vi "Insight_Upgrade.vi"(8 "error in (no error)":errorcluster, 9 "filename":string="?", 10 "Mode (Read / Write)":enum8{"Write", "Read"}(ring), 11 "telnet connection":T1) -> (0 "error out":errorcluster, 1 "upgrade files":string[](array[string]), 2 "response data":string, 3 "telnet  connection out":T1)   [LabVIEW 2015]
uses:
  Telnet Session.ctl
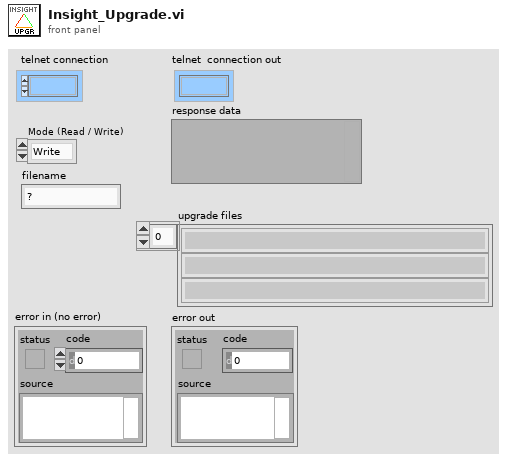
[diagram p1: front panel]
types:
  T1 = typedef "Telnet Session.ctl" = refnum<k1>
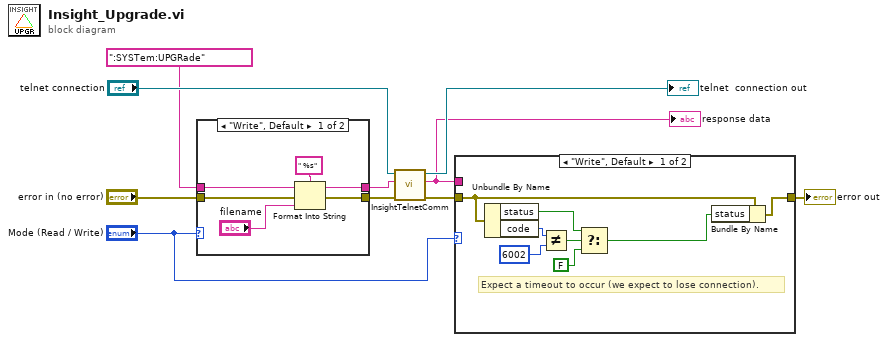
[diagram p0: block diagram]
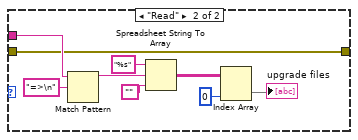
[diagram p2: hidden frame]
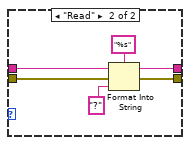
[diagram p3: hidden frame]
diagram:
  n1 = case shown="\"Write\", Default" "Mode (Read / Write)" {
    tunnel: [w12 w18] -> w6
    tunnel: "error in (no error)" -> [w13 w17]
    tunnel: ":SYSTem:UPGRade" ("String") -> [w15 w20]
    tunnel: [w14 w19] -> w5
    frame "Write", Default {
      n2 = Format Into String(format string=" %s", initial string=w15, error in=w13, "filename") -> (resulting string=w14:string, error out=w12:errorcluster)
    }
    frame "Read" {
      n3 = Format Into String(format string="%s", initial string=w20, error in=w17, "?" ("input 1")) -> (resulting string=w19:string, error out=w18:errorcluster)
    }
  }
  n4 = call "InsightTelnetComm.vi"("error in"=w6, "write buffer (\"\")"=w5, "telnet connection"="telnet connection") -> ("error out"=w2:errorcluster, "response data"=w4:string, "telnet  connection out"=→"telnet  connection out":T1)  [unwired: 4 in]
  "response data" <- w4
  n5 = case shown="\"Write\", Default" "Mode (Read / Write)" {
    tunnel: w4 -> [_ w32]
    tunnel: w2 -> [w30 w31]
    tunnel: [w29 w31] -> w1
    frame "Write", Default {
      # "Expect a timeout to occur (we expect to lose connection)."
      n6 = Unbundle By Name(w30) -> ("status"=w25:bool, "code"=w28:i32)
      n7 = Not Equal?(x=w28, y=6002) -> (x != y?=w26:bool)
      n8 = Select(t=w25, s=w26, f=FALSE) -> (s? t:f=w23:bool)
      n9 = Bundle By Name(cluster=w30, "status"=w23) -> (w29:errorcluster)
    }
    frame "Read" {
      n10 = Match Pattern(string=w32, regular expression="=>\n") -> (before substring=w37:string)  [unwired: 1 in, 3 out]
      n11 = Spreadsheet String To Array(format string="%s", spreadsheet string=w37, array type (2D Dbl)="") -> (array=w35:string[][])  [unwired: 1 in]
      n12 = Index Array(array=w35, index (col)=0 ("disabled index (col)")) -> (element=→"upgrade files":string[])  [unwired: 1 in]
    }
  }
  "error out" <- w1
